vi "Arduino_Timed_Release.vi"(2 "Time to hold source ON (microseconds)":u32=100000 format="%.0g", 3 "Time to hold source OFF (microseconds)":u32=1000000 format="%.0g", 4 "Number of cycles":u16=5) -> (0 "error out":errorcluster, 1 "Completed cycles":u16=5)   [LabVIEW 2013]
uses:
  Arduino_comms_Global.vi
panel:
  out "bytes sent":u32=12
  out "write buffer":string
  # "(enter 0 for continuous ON)*"
  # "(enter 0 for continuous OFF)*"
  # "Paul Nathan, 18/06/2013,\n02/05/2014, 12/08/2014"
  # "*until next communication. Ensure n cycles is 1 for these special operations."
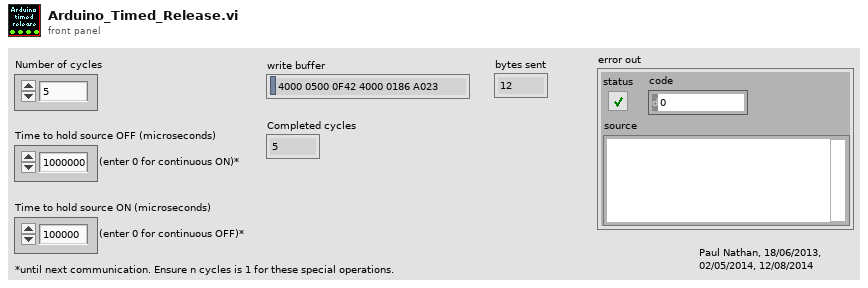
[diagram p1: front panel]
types:
  T1 = typedef "Arduino_comm_params.ctl" = cluster{"VISA resource name":refnum<visa-resource-name>, "byte count":u32, "flow control (0:none)":u16, "stop bits (10: 1 bit)":u16, "parity (0:none)":enum16{"None", "Odd", "Even", "Mark", "Space"}, "data bits (8)":u16, "termination char ":u8, "Enable Termination\nChar":bool, "baud rate (bps)":u32, "timeout (ms)":u32, "Locked":bool}
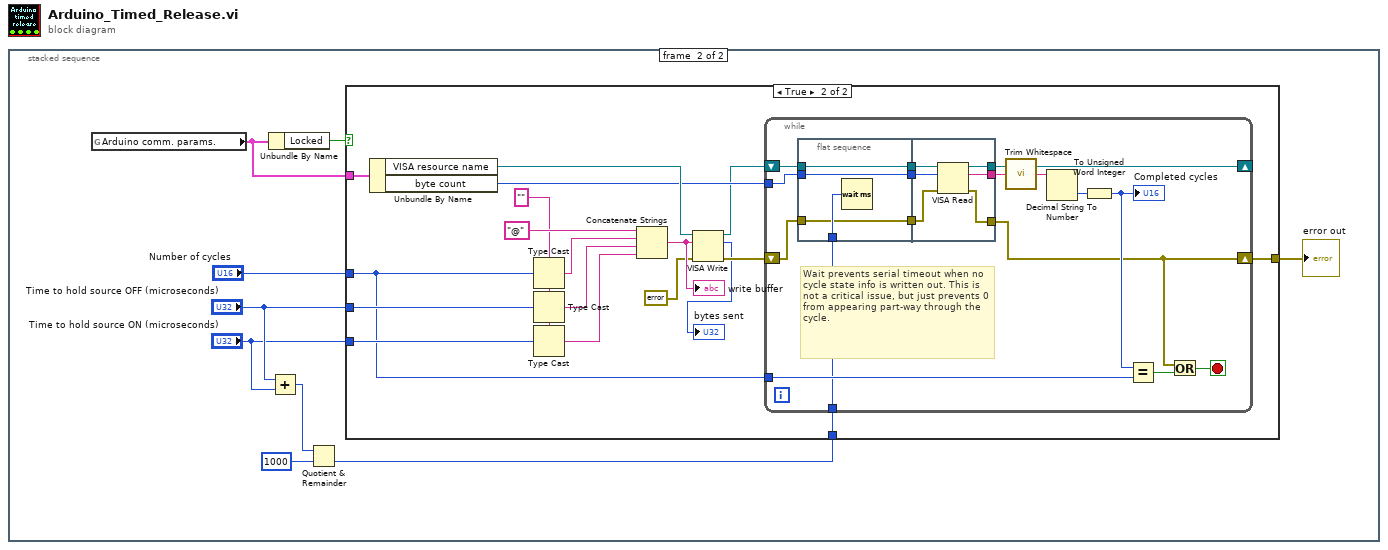
[diagram p0: block diagram]
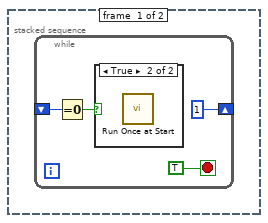
[diagram p2: hidden frame]
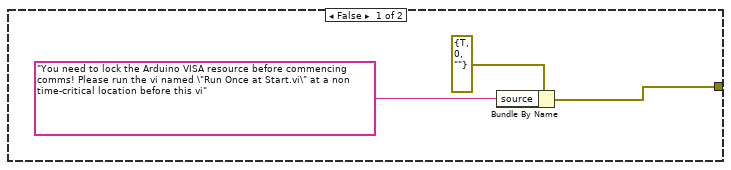
[diagram p4: hidden frame]
diagram:
  n1 = stacked-sequence {
    frame #0 {
      n2 = while {
        shift-right: [1] -> _
        shift-left: _ -> [w4]
        stop <- TRUE stop-if-true
        n3 = Equal To 0?(x=w4) -> (x = 0?=w3:bool)
        n4 = case shown="True" w3 {
          frame False {
          }
          frame True {
            n5 = call "Run Once at Start.vi"() -> ()  [unwired: 1 in]
          }
        }
      }
    }
    frame #1 {
      n6 = global read "Arduino_comms_Global.vi" "Arduino comm. params."() -> (w12:T1)
      n7 = Unbundle By Name(w12) -> ("Locked"=w13:bool)
      n8 = Add(x="Time to hold source OFF (microseconds)", y="Time to hold source ON (microseconds)") -> (x+y=w7:u32)
      n9 = Quotient & Remainder(x=w7, y=u32 1000) -> (floor(x/y)=w5:u32)  [unwired: 1 out]
      n10 = case shown="True" w13 {
        tunnel: w12 -> [_ w32]
        tunnel: "Number of cycles" -> [_ w20]
        tunnel: "Time to hold source OFF (microseconds)" -> [_ w30]
        tunnel: "Time to hold source ON (microseconds)" -> [_ w29]
        tunnel: [w14 w22] -> w10
        tunnel: w5 -> [_ w17]
        frame False {
          n11 = Bundle By Name(cluster=errorcluster {"status"=TRUE, "code"=0, "source"=""} ("error out"), "source"="You need to lock the Arduino VISA resource before commencing comms! Please run the vi named \"Run Once at Start.vi\" at a non time-critical location before this vi") -> (w14:errorcluster)
        }
        frame True {
          w31 = ""
          n12 = Unbundle By Name(w32) -> ("VISA resource name"=w25:refnum<visa-resource-name>, "byte count"=w24:u32)
          n13 = Type Cast(type=w31, x=w20) -> (*(type *) &x=w28:string)
          n14 = Type Cast(type=w31, x=w30) -> (*(type *) &x=w27:string)
          n15 = Type Cast(type=w31, x=w29) -> (*(type *) &x=w26:string)
          n16 = Concatenate Strings("@", w28, w27, w26) -> (w33:string)
          "write buffer" <- w33
          n17 = VISA Write(VISA resource name=w25, write buffer=w33, error in (no error)=errorcluster {"status"=FALSE, "code"=0, "source"=""}) -> (VISA resource name out=w19:refnum<visa-resource-name>, return count=→"bytes sent":u32, error out=w23:errorcluster)
          n18 = while {
            tunnel: w24 -> [w49]
            shift-right: [w37] -> w22
            shift-left: w23 -> [w39]
            shift-right: [w48] -> _
            shift-left: w19 -> [w50]
            tunnel: w20 -> [w46]
            tunnel: w17 -> [w40]
            stop <- w35 stop-if-true
            # "Wait prevents serial timeout when no cycle state info is written out. This is not a critical issue, but just prevents 0 from appearing part-way through the cycle."
            n19 = flat-sequence {
              tunnel: w49 -> [w53]
              tunnel: w50 -> [w54]
              tunnel: [w54] -> w42
              tunnel: [w53] -> w41
              tunnel: w40 -> [w52]
              tunnel: w39 -> [w51]
              tunnel: [w51] -> w38
              tunnel: [w58] -> w48
              tunnel: [w57] -> w44
              tunnel: w42 -> [w60]
              tunnel: w41 -> [w59]
              tunnel: w38 -> [w56]
              tunnel: [w55] -> w37
              frame #0 {
                n20 = Wait (ms)(milliseconds to wait=w52) -> ()  [unwired: 1 out]
              }
              frame #1 {
                n21 = VISA Read(VISA resource name=w60, byte count=w59, error in (no error)=w56) -> (VISA resource name out=w58:refnum<visa-resource-name>, read buffer=w57:string, error out=w55:errorcluster)  [unwired: 1 out]
              }
            }
            n22 = call <vilib>:"Trim Whitespace.vi"("string"=w44) -> ("trimmed string"=w43:string)  [unwired: 1 in]
            n23 = Decimal String To Number(string=w43) -> (number=w47:i32)  [unwired: 2 in, 1 out]
            n24 = To Unsigned Word Integer(number=w47) -> (unsigned 16bit integer=w45:u16)
            "Completed cycles" <- w45
            n25 = Equal?(x=w45, y=w46) -> (x = y?=w36:bool)
            n26 = Or(x=w37, y=w36) -> (x .or. y?=w35:bool)
          }
        }
      }
      "error out" <- w10
    }
  }
